vi "GetPointType2D_4D-I32.vi"(11 "Point":T1) -> (3 "Point":T2)   [LabVIEW 2020, in "OpenLvVision_OpenCv.lvlib"]
uses:
  TypeDef/Point/2D_PointI32.ctl
  OpenLvVision_OpenCv.lvlib
  TypeDef/Point/4D_PointI32.ctl
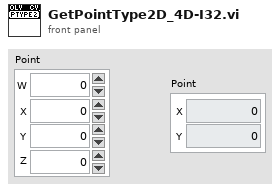
[diagram p1: front panel]
types:
  T1 = typedef "OpenLvVision_OpenCv.lvlib/4D_PointI32.ctl" = cluster{"W":i32, "X":i32, "Y":i32, "Z":i32}
  T2 = typedef "OpenLvVision_OpenCv.lvlib/2D_PointI32.ctl" = cluster{"X":i32, "Y":i32}
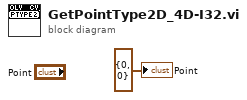
[diagram p0: block diagram]
diagram:
  "Point" <- T2 {"X"=0, "Y"=0} ("Point")
